vi "usuń ogon.vi"(8 "Po ogonie?":bool, 9 "ogon":T1[](array[typedef]), 10 "Array 3":dbl[][](array[numeric]), 11 "zjadł?":bool) -> (2 "ogon":T1[](array[typedef]), 3 "Array 2":dbl[][](array[numeric]))   [LabVIEW 2020]
uses:
  <vilib>/event_ctls.llb/eventvkey.ctl
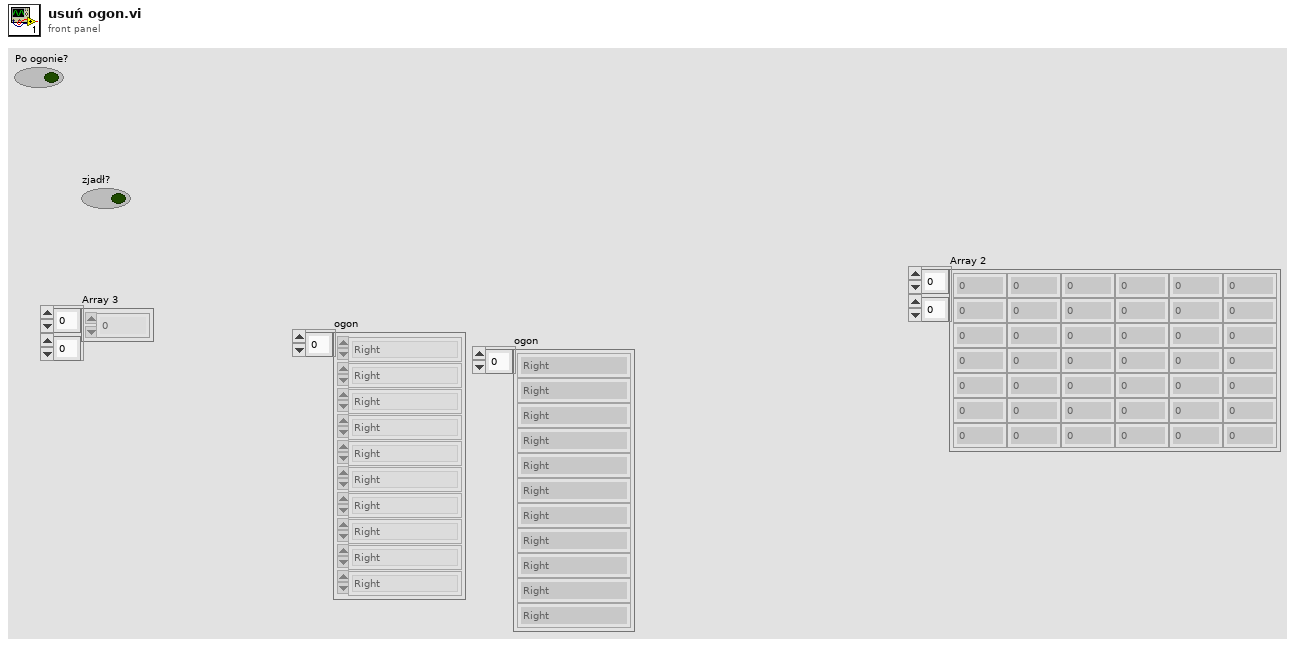
[diagram p1: front panel]
types:
  T1 = typedef "eventvkey.ctl" = enum16{"ASCII", "Enter", "Return", "Shift", "Ctrl", "Alt", "Cmd", "Opt", "Caps", "NumLock", "Clear", "Break", "Up", "Down", "Left", "Right", "Insert", "Delete", "Home", "End", "PageUp", "PageDown", "Escape", "Help", "Pause", "ScrollLock", "F1", "F2", "F3", "F4", "F5", "F6", "F7", "F8", "F9", "F10", "F11", "F12", "F13", "F14", "F15", "F16", "F17", "F18", "F19", "F20", "F21", "F22", "F23", "F24", "Play", "VolumeUp", "VolumeDown", "Mute", "Two Byte Char"}
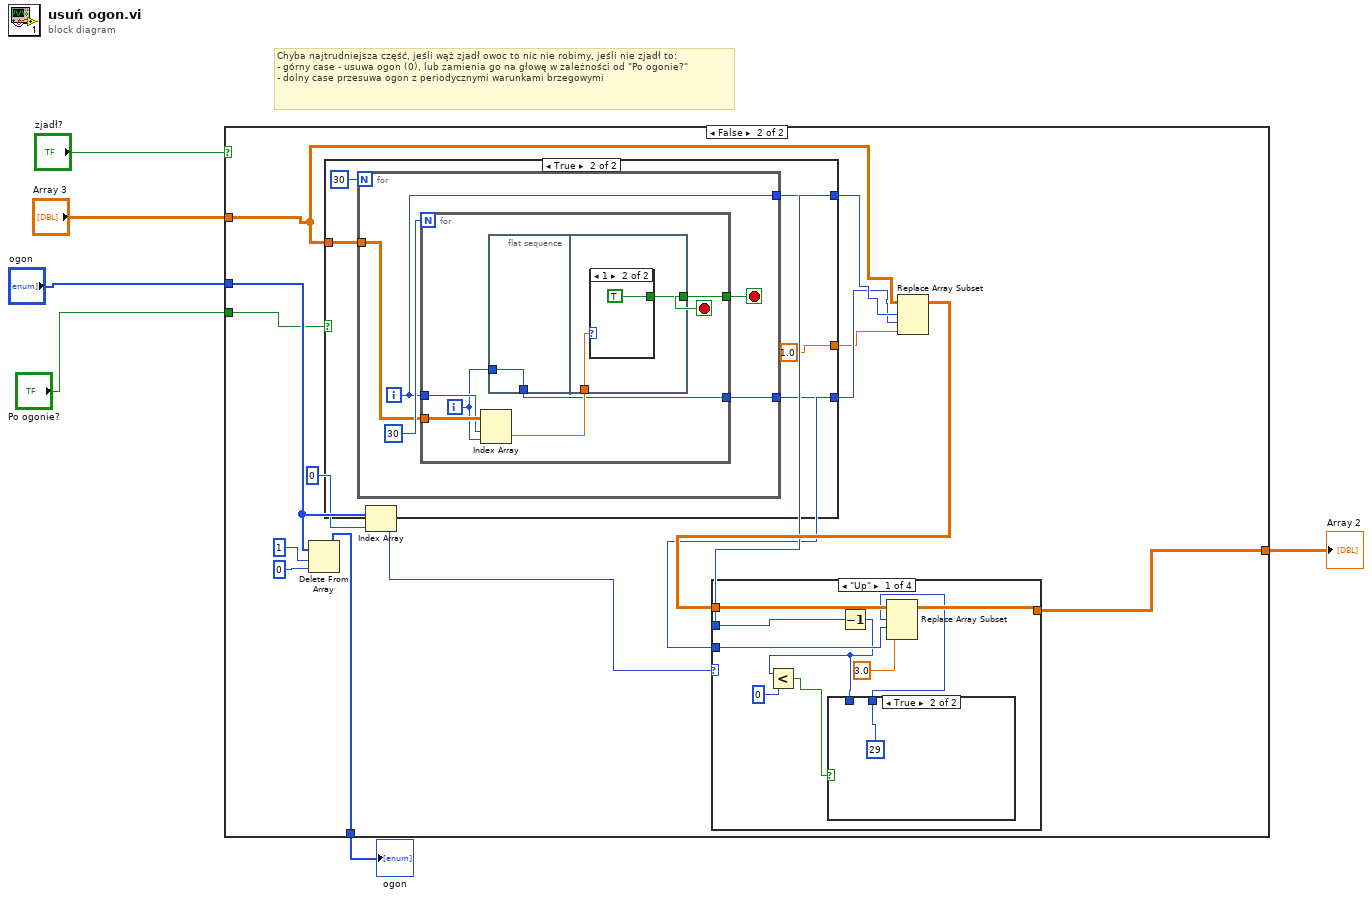
[diagram p0: block diagram]
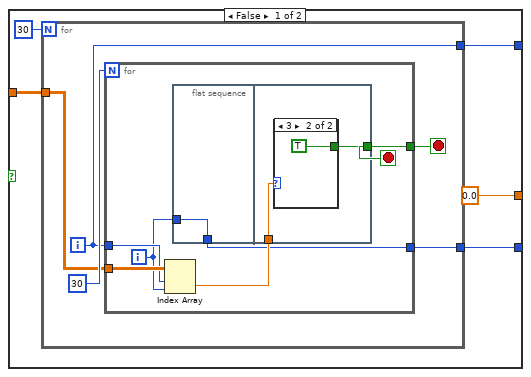
[diagram p3: hidden frame]
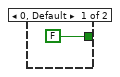
[diagram p4: hidden frame]
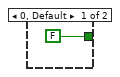
[diagram p5: hidden frame]
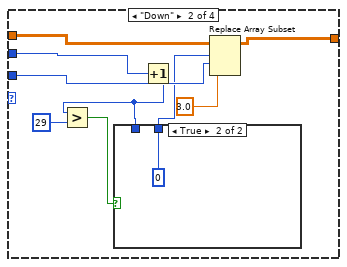
[diagram p7: hidden frame]
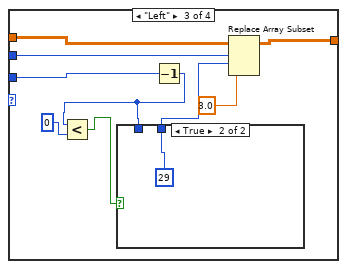
[diagram p9: hidden frame]
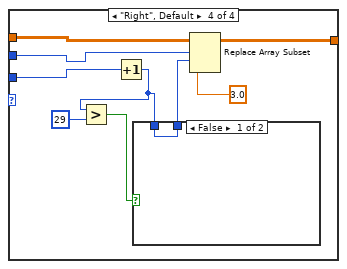
[diagram p11: hidden frame]
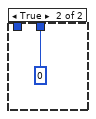
[diagram p12: hidden frame]
diagram:
  # "Chyba najtrudniejsza część, jeśli wąż zjadł owoc to nic nie robimy, jeśli nie zjadł to:\n- górny case - usuwa ogon (0), lub zamienia go na głowę w zależności od \"Po ogonie?\"\n- dolny case przesuwa ogon z periodycznymi warunkami brzegowymi"
  n1 = case shown="False" "zjadł?" {
    tunnel: "Array 3" -> [w8 w18]
    tunnel: [w8 w11] -> w5
    tunnel: "ogon" -> [w7 w17]
    tunnel: [w7 w19] -> w2
    tunnel: "Po ogonie?" -> [_ w10]
    frame True {
    }
    frame False {
      n2 = Delete From Array(array=w17, length=1, index=0) -> (array with subset deleted=w19:T1[])  [unwired: 1 out]
      n3 = case shown="True" w10 {
        tunnel: w18 -> [w26 w47]
        tunnel: [w24 w45] -> w13
        tunnel: [w23 w44] -> w12
        tunnel: [0.0 ("new element/subarray") 1.0 ("new element/subarray")] -> w9
        frame False {
          n4 = for {
            N: 30 -> [_]
            tunnel: w26 -> [w30]
            tunnel: [w29] -> w23
            tunnel: [w28] -> w24
            i -> [w28]
            stop <- w27 stop-if-true
            n5 = for {
              N: 30 -> [_]
              tunnel: w30 -> [w37]
              tunnel: w28 -> [w36]
              tunnel: [w33] -> w29
              tunnel: [w32] -> w27
              i -> [w34]
              stop <- w32 stop-if-true
              n6 = Index Array(array=w37, index (row)=w36, index (col)=w34) -> (element=w35:dbl)
              n7 = flat-sequence {
                tunnel: w34 -> [w38]
                tunnel: [w38] -> w33
                tunnel: w35 -> [w40]
                tunnel: [w39] -> w32
                frame #0 {
                }
                frame #1 {
                  n8 = case shown="3" w40 {
                    tunnel: [FALSE TRUE] -> w39
                    frame 0, Default {
                    }
                    frame 3 {
                    }
                  }
                }
              }
            }
          }
        }
        frame True {
          n9 = for {
            N: 30 -> [_]
            tunnel: w47 -> [w51]
            tunnel: [w50] -> w44
            tunnel: [w49] -> w45
            i -> [w49]
            stop <- w48 stop-if-true
            n10 = for {
              N: 30 -> [_]
              tunnel: w51 -> [w58]
              tunnel: w49 -> [w57]
              tunnel: [w54] -> w50
              tunnel: [w53] -> w48
              i -> [w55]
              stop <- w53 stop-if-true
              n11 = Index Array(array=w58, index (row)=w57, index (col)=w55) -> (element=w56:dbl)
              n12 = flat-sequence {
                tunnel: w55 -> [w59]
                tunnel: [w59] -> w54
                tunnel: w56 -> [w61]
                tunnel: [w60] -> w53
                frame #0 {
                }
                frame #1 {
                  n13 = case shown="1" w61 {
                    tunnel: [FALSE TRUE] -> w60
                    frame 0, Default {
                    }
                    frame 1 {
                    }
                  }
                }
              }
            }
          }
        }
      }
      n14 = Index Array(array=w17, index=0) -> (element=w15:T1)
      n15 = Replace Array Subset(array=w18, new element=w9, index (row)=w13, index (col)=w12) -> (w14:dbl[][])
      n16 = case shown="\"Up\"" w15 {
        tunnel: w14 -> [w72 w82 w93 w104]
        tunnel: w13 -> [w71 w80 w90 w101]
        tunnel: w12 -> [w70 w81 w91 w102]
        tunnel: [w68 w79 w92 w103] -> w11
        frame "Up" {
          n17 = Decrement(x=w71) -> (x-1=w65:i32)
          n18 = Less?(x=w65, y=0) -> (x < y?=w66:bool)
          n19 = case shown="True" w66 {
            tunnel: w65 -> [w73 _]
            tunnel: [w73 29] -> w64
            frame False {
            }
            frame True {
            }
          }
          n20 = Replace Array Subset(array=w72, new element=3.0 ("new element/subarray"), index (row)=w64, index (col)=w70) -> (w68:dbl[][])
        }
        frame "Down" {
          n21 = Increment(x=w80) -> (x+1=w76:i32)
          n22 = Greater?(x=w76, y=29) -> (0:w77:bool)
          n23 = case shown="True" w77 {
            tunnel: w76 -> [w84 _]
            tunnel: [w84 0] -> w75
            frame False {
            }
            frame True {
            }
          }
          n24 = Replace Array Subset(array=w82, new element=3.0 ("new element/subarray"), index (row)=w75, index (col)=w81) -> (w79:dbl[][])
        }
        frame "Left" {
          n25 = Decrement(x=w91) -> (x-1=w88:i32)
          n26 = Less?(x=w88, y=0) -> (x < y?=w86:bool)
          n27 = case shown="True" w86 {
            tunnel: w88 -> [w95 _]
            tunnel: [w95 29] -> w89
            frame False {
            }
            frame True {
            }
          }
          n28 = Replace Array Subset(array=w93, new element=3.0 ("new element/subarray"), index (row)=w90, index (col)=w89) -> (w92:dbl[][])
        }
        frame "Right", Default {
          n29 = Increment(x=w102) -> (x+1=w98:i32)
          n30 = Greater?(x=w98, y=29) -> (0:w99:bool)
          n31 = case shown="False" w99 {
            tunnel: w98 -> [w106 _]
            tunnel: [w106 0] -> w97
            frame False {
            }
            frame True {
            }
          }
          n32 = Replace Array Subset(array=w104, new element=3.0 ("new element/subarray"), index (row)=w101, index (col)=w97) -> (w103:dbl[][])
        }
      }
    }
  }
  "Array 2" <- w5
  "ogon" <- w2
